vi "Move Scan frame to new coords.vi"(0 "Dx, Dy":cluster{"Xc":sgl, "Yc":sgl}={"Xc"=nan, "Yc"=nan} caption="Drift  (m) (NaN=no change)" {"Yc" format="%.2p"; "Xc" format="%.2p"}) -> (7 "Corrected Coordinates":cluster{"Initial x":dbl, "Initial y":dbl}, 10 "error out":errorcluster)   [LabVIEW 2025]
uses:
  <userlib>/Nanonis Prog Interface V5e/Nanonis Prog Interface.lvlib
panel:
  out "Inital Coordinates (m)":cluster{"Xc":sgl, "Yc":sgl} {"Yc" format="%.2p"; "Xc" format="%.2p"}
  out "Dx, Dy 2":cluster{"Xc":sgl, "Yc":sgl}={"Xc"=nan, "Yc"=nan} caption="Drift (m) (NaN=no change)" {"Yc" format="%.2p"; "Xc" format="%.2p"}
  out "Xc":sgl
  out "Yc":sgl
  in  "Port number (3364)":u32=3364
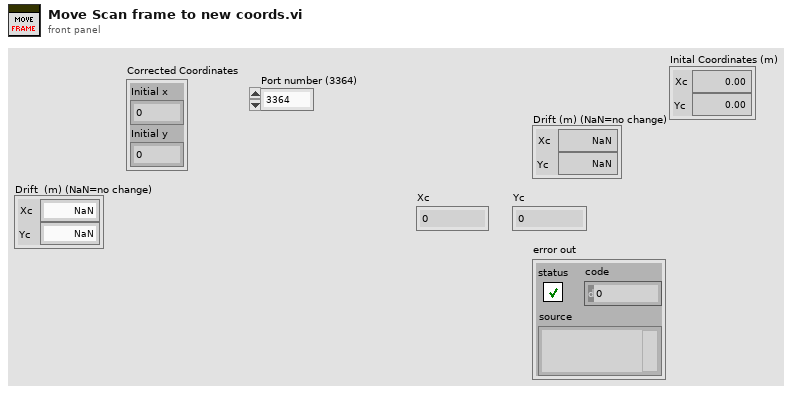
[diagram p1: front panel]
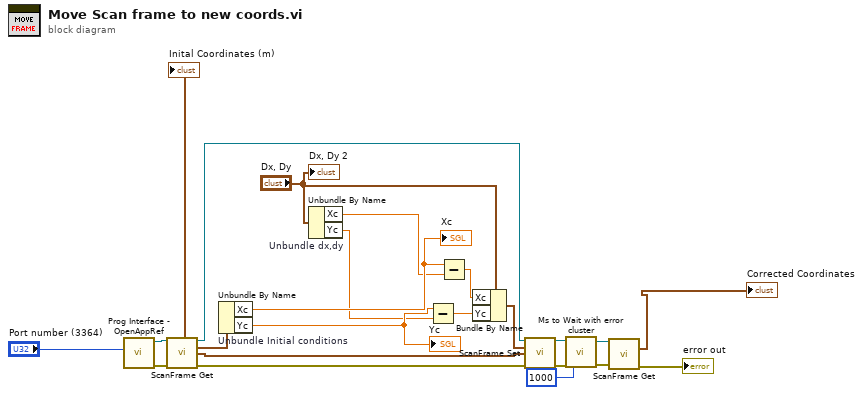
[diagram p0: block diagram]
diagram:
  n1 = call <userlib>:"Prog Interface - OpenAppRef.vi"("Port number (3364)"="Port number (3364)") -> ("Error out"=w18:errorcluster, "Application reference"=w17:refnum<vi>)  [unwired: 5 in]
  n2 = call <userlib>:"ScanFrame Get.vi"("Application ref in"=w17, "error in (no error)"=w18) -> ("Application ref out"=w16:refnum<vi>, "Center coordinates (m)"=w4:cluster{"Xc":sgl, "Yc":sgl}, "Size (m)"=w8:cluster{"Width":sgl, "Height":sgl}, "error out"=w15:errorcluster)  [unwired: 9 in, 1 out]
  "Inital Coordinates (m)" <- w4
  n3 = Unbundle By Name "Unbundle Initial conditions"(w4) -> ("Xc"=w14:sgl, "Yc"=w7:sgl)
  "Yc" <- w7
  "Xc" <- w14
  n4 = Unbundle By Name "Unbundle dx,dy"("Dx, Dy") -> ("Xc"=w13:sgl, "Yc"=w6:sgl)
  n5 = Subtract(x=w7, y=w6) -> (x-y=w9:sgl)
  n6 = Subtract(x=w14, y=w13) -> (x-y=w10:sgl)
  n7 = Bundle By Name(cluster="Dx, Dy", "Xc"=w10, "Yc"=w9) -> (w11:cluster{"Xc":sgl, "Yc":sgl})
  n8 = call <userlib>:"ScanFrame Set.vi"("Application ref in"=w16, "Center coordinates (m)"=w11, "Size (m)"=w8, "error in (no error)"=w15) -> ("Application ref out"=w21:refnum<vi>, "error out"=w3:errorcluster)  [unwired: 10 in]
  n9 = call <userlib>:"Ms to Wait with error cluster.vi"("error in (no error)"=w3, "milliseconds to wait"=u32 1000) -> ("error out"=w2:errorcluster)  [unwired: 4 in, 1 out]
  n10 = call <userlib>:"ScanFrame Get.vi"("Application ref in"=w21, "error in (no error)"=w2) -> ("Center coordinates (m)"=→"Corrected Coordinates":cluster{"Xc":sgl, "Yc":sgl}, "error out"=→"error out":errorcluster)  [unwired: 9 in, 3 out]
  "Dx, Dy 2" <- "Dx, Dy"
